vi "relay board with toggle switch array.vi"() -> ()   [LabVIEW 2013]
panel:
  in  "Relays":bool[](array[boolean])
  out "Waveform Chart":dynamicdata(graph) caption="Voltage"
  out "Output":dbl
  out "Input":dbl
  in  "Slide":dbl(slide) scale=-10.0..10.0
  in  "stop":bool
  # "69"
  # "70"
  # "71"
  # "72"
  # "65"
  # "66"
  # "67"
  # "68"
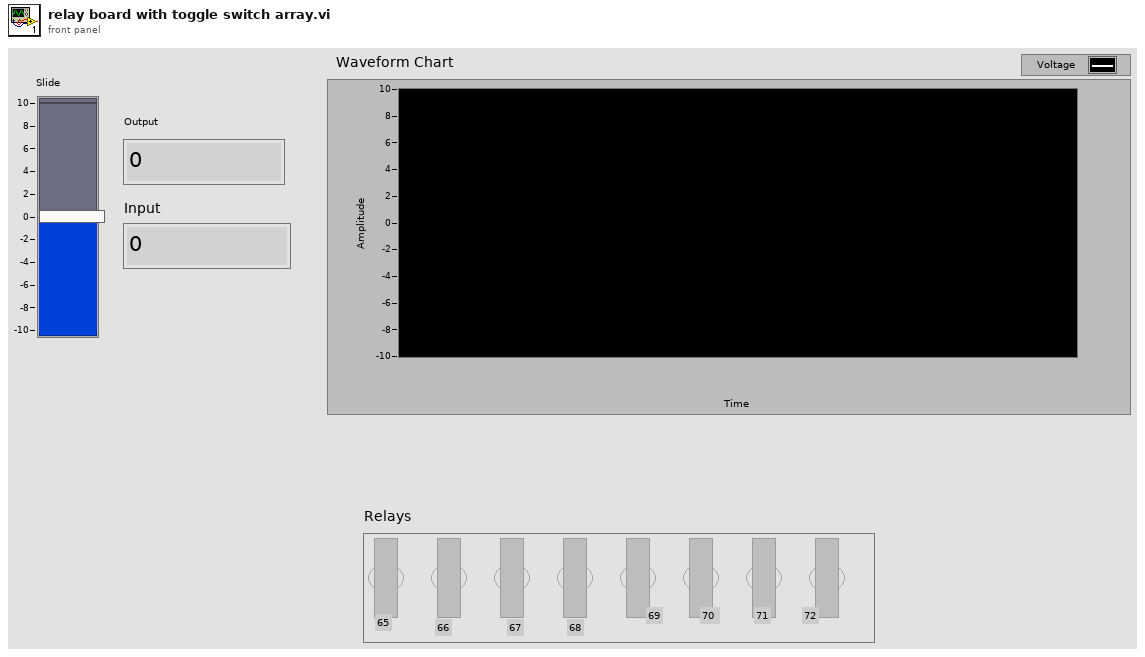
[diagram p1: front panel]
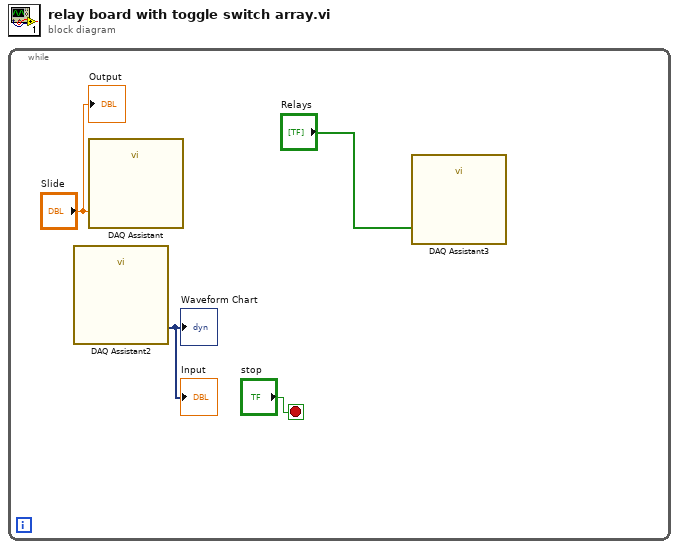
[diagram p0: block diagram]
diagram:
  n1 = while {
    stop <- "stop" stop-if-true
    n2 = call "DAQ Assistant2"() -> ("data"=→"Input" →"Waveform Chart":dynamicdata)  [unwired: 16 in, 3 out]
    n3 = call "DAQ Assistant"("data"="Slide") -> ()  [unwired: 17 in, 2 out]
    n4 = call "DAQ Assistant3"("data"="Relays") -> ()  [unwired: 17 in, 2 out]
    "Output" <- "Slide"
  }
